vi "Target Logging Detection.vi"(8 "Main Clock Line (s)":dbl, 9 "Vicon Logging Signal":dbl, 11 "Trigger High?":bool) -> (3 "Valid for Logging?":bool)   [LabVIEW 2018]
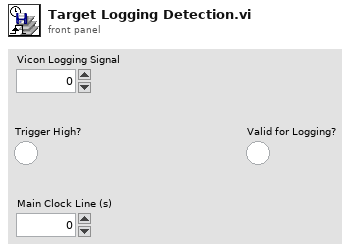
[diagram p1: front panel]
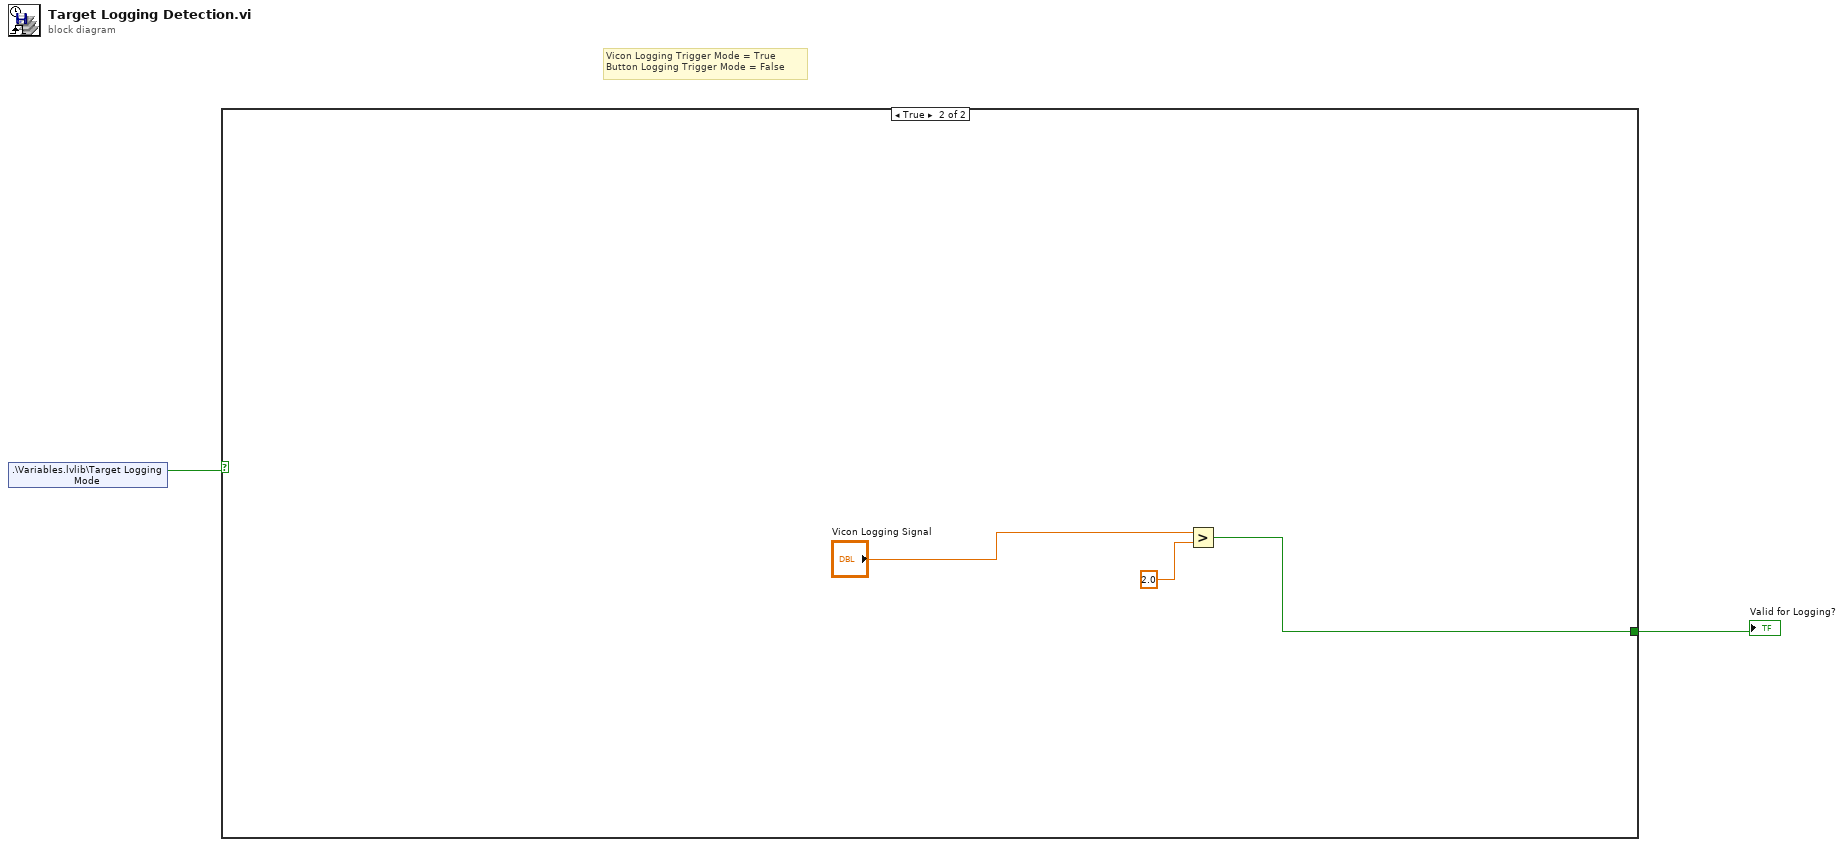
[diagram p0: block diagram]
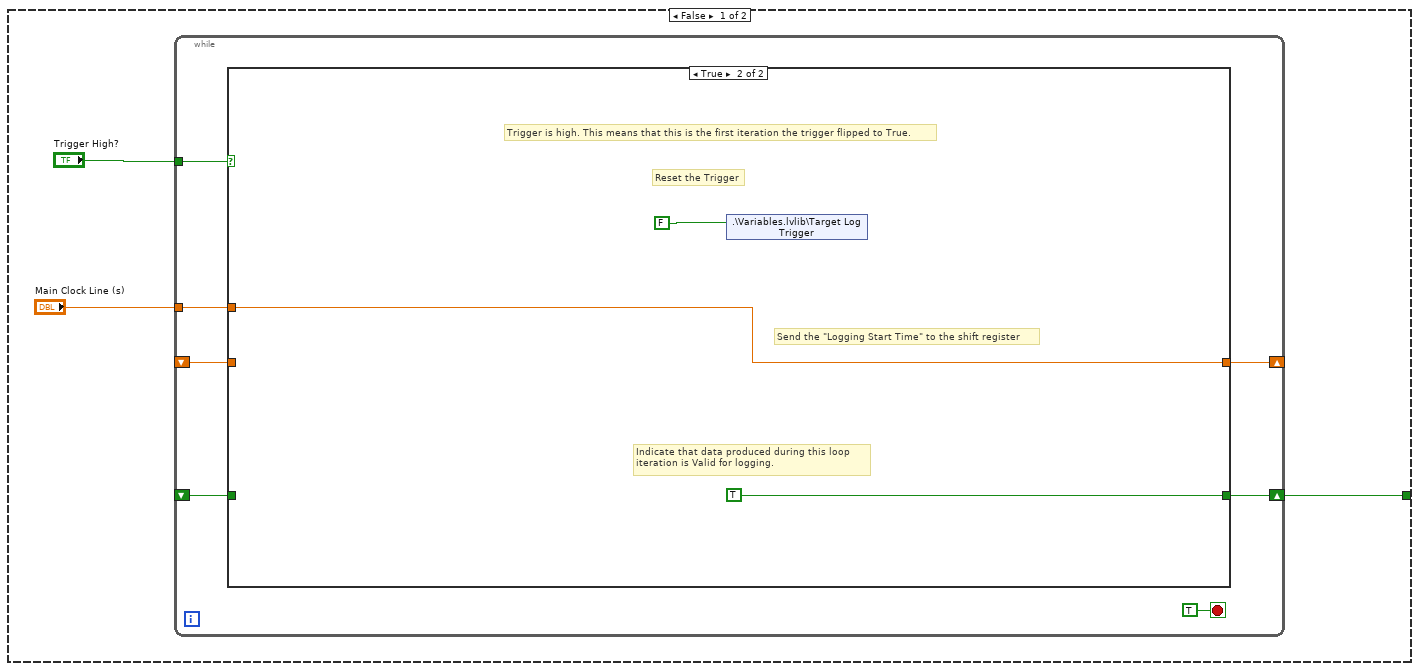
[diagram p2: hidden frame]
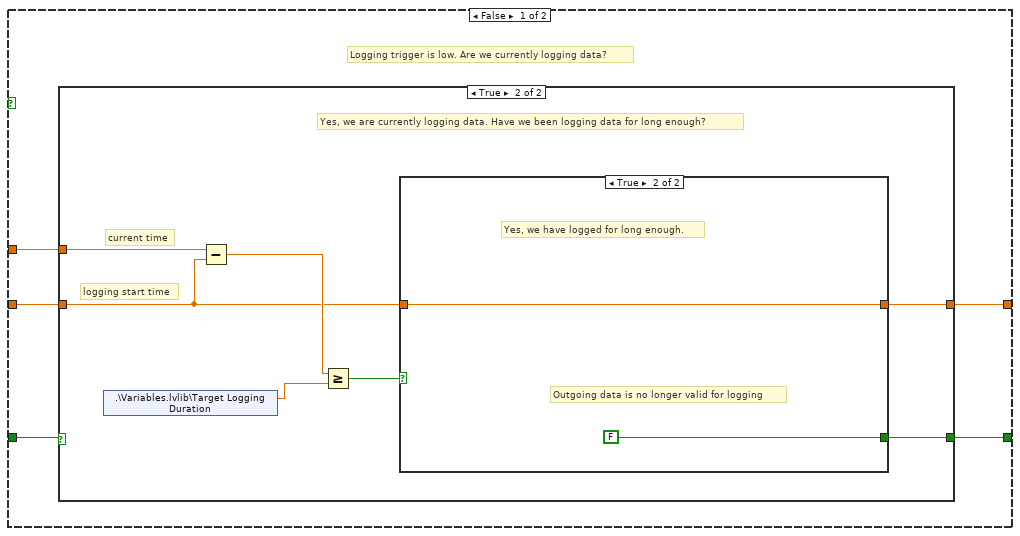
[diagram p3: hidden frame]
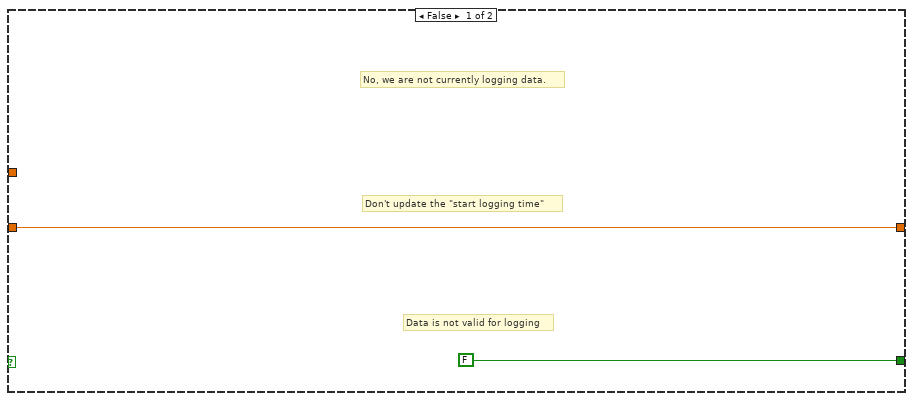
[diagram p4: hidden frame]
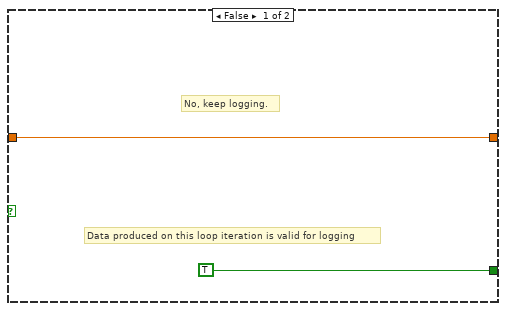
[diagram p5: hidden frame]
diagram:
  # "Vicon Logging Trigger Mode = True\nButton Logging Trigger Mode = False"
  n1 = shared-variable ".\\Variables.lvlib\\Target Logging Mode"() -> (w1:bool)  [unwired: 1 in, 1 out]
  n2 = case shown="True" w1 {
    tunnel: [w4 w35] -> w2
    frame False {
      n3 = while {
        tunnel: "Trigger High?" -> [w11]
        shift-right: [w10] -> w4
        shift-left: _ -> [w8]
        shift-right: [w9] -> _
        shift-left: _ -> [w7]
        tunnel: "Main Clock Line (s)" -> [w6]
        stop <- TRUE stop-if-true
        n4 = case shown="True" w11 {
          tunnel: [w15 TRUE] -> w10
          tunnel: [w16 w32] -> w9
          tunnel: w8 -> [w17 _]
          tunnel: w7 -> [w14 _]
          tunnel: w6 -> [w13 w32]
          frame False {
            # "Logging trigger is low. Are we currently logging data?"
            n5 = case shown="True" w17 {
              tunnel: [w18 w25] -> w16
              tunnel: [FALSE w24] -> w15
              tunnel: w14 -> [w18 w20]
              tunnel: w13 -> [_ w23]
              frame False {
                # "Data is not valid for logging"
                # "Don't update the \"start logging time\""
                # "No, we are not currently logging data."
              }
              frame True {
                # "logging start time"
                # "current time"
                # "Yes, we are currently logging data. Have we been logging data for long enough?"
                n6 = shared-variable ".\\Variables.lvlib\\Target Logging Duration"() -> (w22:dbl)  [unwired: 1 in, 1 out]
                n7 = Subtract(x=w23, y=w20) -> (x-y=w21:dbl)
                n8 = Greater Or Equal?(x=w21, y=w22) -> (x >= y?=w26:bool)
                n9 = case shown="True" w26 {
                  tunnel: [w27 w29] -> w25
                  tunnel: [TRUE FALSE] -> w24
                  tunnel: w20 -> [w27 w29]
                  frame False {
                    # "Data produced on this loop iteration is valid for logging"
                    # "No, keep logging."
                  }
                  frame True {
                    # "Outgoing data is no longer valid for logging"
                    # "Yes, we have logged for long enough."
                  }
                }
              }
            }
          }
          frame True {
            # "Indicate that data produced during this loop\niteration is Valid for logging."
            # "Send the \"Logging Start Time\" to the shift register"
            # "Reset the Trigger"
            # "Trigger is high. This means that this is the first iteration the trigger flipped to True."
            n10 = shared-variable ".\\Variables.lvlib\\Target Log Trigger"(FALSE ("PXI Log Trigger")) -> ()  [unwired: 1 in, 1 out]
          }
        }
      }
    }
    frame True {
      n11 = Greater?(x="Vicon Logging Signal", y=2.0) -> (0:w35:bool)
    }
  }
  "Valid for Logging?" <- w2
